vi "ExposeConnect.vi"(8 "error in (no error)":errorcluster, 11 "Expose Info":T1) -> (0 "error out":errorcluster, 3 "Expose Info out":T1)   [LabVIEW 2017]
uses:
  ExposeInfo.ctl
  C:/Code/CMCryoSysCode/Expose/COM/CSCom/CSCom/bin/Release/CSCom.dll
  COM/CSCom/CSCom/bin/Release/CSCom.dll
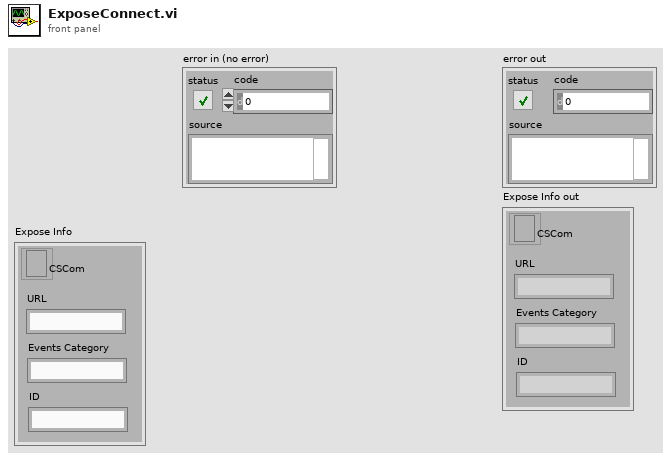
[diagram p1: front panel]
types:
  T1 = typedef "ExposeInfo.ctl" = cluster{"CSCom":refnum<k24>, "URL":string, "Events Category":string, "ID":string}
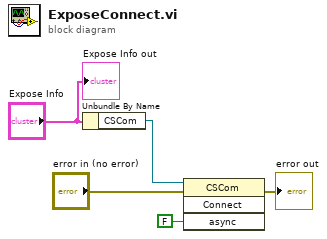
[diagram p0: block diagram]
diagram:
  n1 = Unbundle By Name("Expose Info") -> ("CSCom"=w1:refnum<k24>)
  n2 = invoke class="CSCom" method="Connect"(reference=w1, error in="error in (no error)", "async"=FALSE) -> (error out=→"error out":errorcluster)  [unwired: 1 in, 3 out]
  "Expose Info out" <- "Expose Info"
